vi "Write Childs Subpanel.vi"(8 "error in (no error)":errorcluster, 10 "Childs Subpanel":refnum<vi>, 11 "ViewableActorEncaps in":refnum<class "ViewableActorEncaps.lvclass">) -> (0 "error out":errorcluster, 3 "ViewableActorEncaps out":refnum<class "ViewableActorEncaps.lvclass">)   [LabVIEW 2020, in "ViewableActor.lvlib" / "ViewableActorEncaps.lvclass"]
uses:
  ViewableActorEncaps.lvclass
  ViewableActorEncaps.lvclass/ViewableActorEncaps.ctl
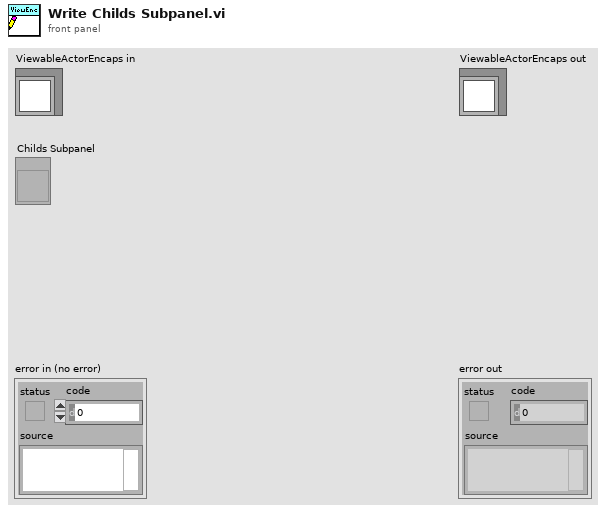
[diagram p1: front panel]
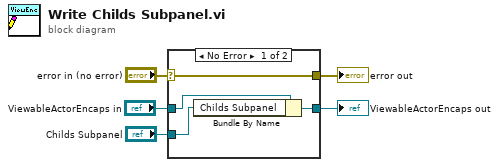
[diagram p0: block diagram]
diagram:
  n1 = case shown="No Error" "error in (no error)" {
    selector: "error in (no error)" -> [w9 w10]
    tunnel: [w9 w10] -> w4
    tunnel: [w7 w11] -> w2
    tunnel: "ViewableActorEncaps in" -> [w8 w11]
    tunnel: "Childs Subpanel" -> [w6 _]
    frame No Error {
      n2 = Bundle By Name(cluster=w8, "Childs Subpanel"=w6) -> (w7:refnum<class "ViewableActorEncaps.lvclass">)
    }
    frame Error {
    }
  }
  "error out" <- w4
  "ViewableActorEncaps out" <- w2
